vi "port Handler.vi"(11 "port_name":string) -> (3 "function return":i32)   [LabVIEW 2015, in "dxl_x86_c.lvlib"]
doc: "WINDECLSPEC int portHandler (const char *port_name);"
uses:
  dxl_x86_c.lvlib
  dxl_x86_c.dll
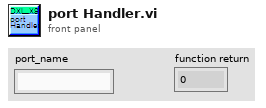
[diagram p1: front panel]
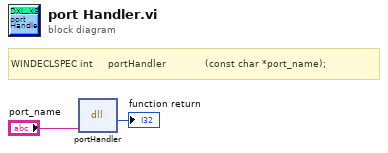
[diagram p0: block diagram]
diagram:
  # "WINDECLSPEC int     portHandler             (const char *port_name);"
  n1 = dll-call lib="C:/Users/Platform/Desktop/LabVIEW/dxl_x86_c.lvlib/dxl_x86_c.*" fn="portHandler"("port_name"="port_name") -> (→"function return":i32)  [unwired: 4 in, 2 out]
